vi "Periodic Tasks.vi"(8 "error in":errorcluster) -> ()   [LabVIEW 2023]
doc: "This VI runs in parallel to other robot code. It can contain as many user-defined periodic loops as you need. These can carry out PID or other sorts of timed response."
uses:
  <vilib>/Rock Robotics/WPI/Joystick/XBox Buttons Indexer.ctl
  AimTIFKATS/Implementation/AimTIFKATS Operations.ctl
  Undertake/Implementation/Undertake Operations.ctl
  TIFKATS/Implementation/TIFKATS Operations.ctl
  <vilib>/Rock Robotics/WPI/Utilities/WPI_GetSetVariantRefNum.vi
  <vilib>/Rock Robotics/Network Tables/NT Write Boolean.vi
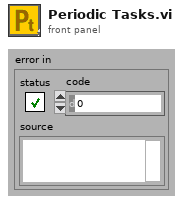
[diagram p1: front panel]
types:
  T1 = typedef "WPI_JoystickDevRef.ctl" = cluster{"Device":T2}
  T2 = typedef "WPI_JoystickDeviceEnum.ctl" = enum16{"USB 0", "USB 1", "USB 2", "USB 3", "USB 4", "USB 5"}
  T3 = typedef "XBox Buttons Indexer.ctl" = enum16{"A", "B", "X", "Y", "Left Bumper", "Right Bumper", "Back", "Start", "Left Joystick", "Right Joystick"}
  T4 = typedef "Undertake Operations.ctl" = enum16{"Reserve", "Read Current", "Immediate", "Onn", "Offf", "Reject"}
  T5 = typedef "AimTIFKATS Operations.ctl" = enum16{"Reserve", "Read Current", "Immediate", "Angle up", "Angle down", "Angle to angle", "Stop rotate"}
  T6 = typedef "TIFKATS Operations.ctl" = enum16{"Reserve", "Read Current", "Immediate", "Load", "Shoot", "Intake", "Spit", "Stop All"}
  T7 = typedef "WPI_DigitalInputDevRef.ctl" = cluster{"DevStatus":errorcluster, "DIO Channel":T8}
  T8 = typedef "FPGA_DIOChannel.ctl" = enum8{"DIO 0", "DIO 1", "DIO 2", "DIO 3", "DIO 4", "DIO 5", "DIO 6", "DIO 7", "DIO 8", "DIO 9", "DIO MXP 0", "DIO MXP 1", "DIO MXP 2", "DIO MXP 3", "DIO MXP 4", "DIO MXP 5", "DIO MXP 6", "DIO MXP 7", "DIO MXP 8", "DIO MXP 9", "DIO MXP 10", "DIO MXP 11", "DIO MXP 12", "DIO MXP 13", "DIO MXP 14", "DIO MXP 15", "SPI Port CS1", "SPI Port CS2", "SPI Port CS3", "SPI Port MISO", "SPI Port MOSI", "Invalid"}
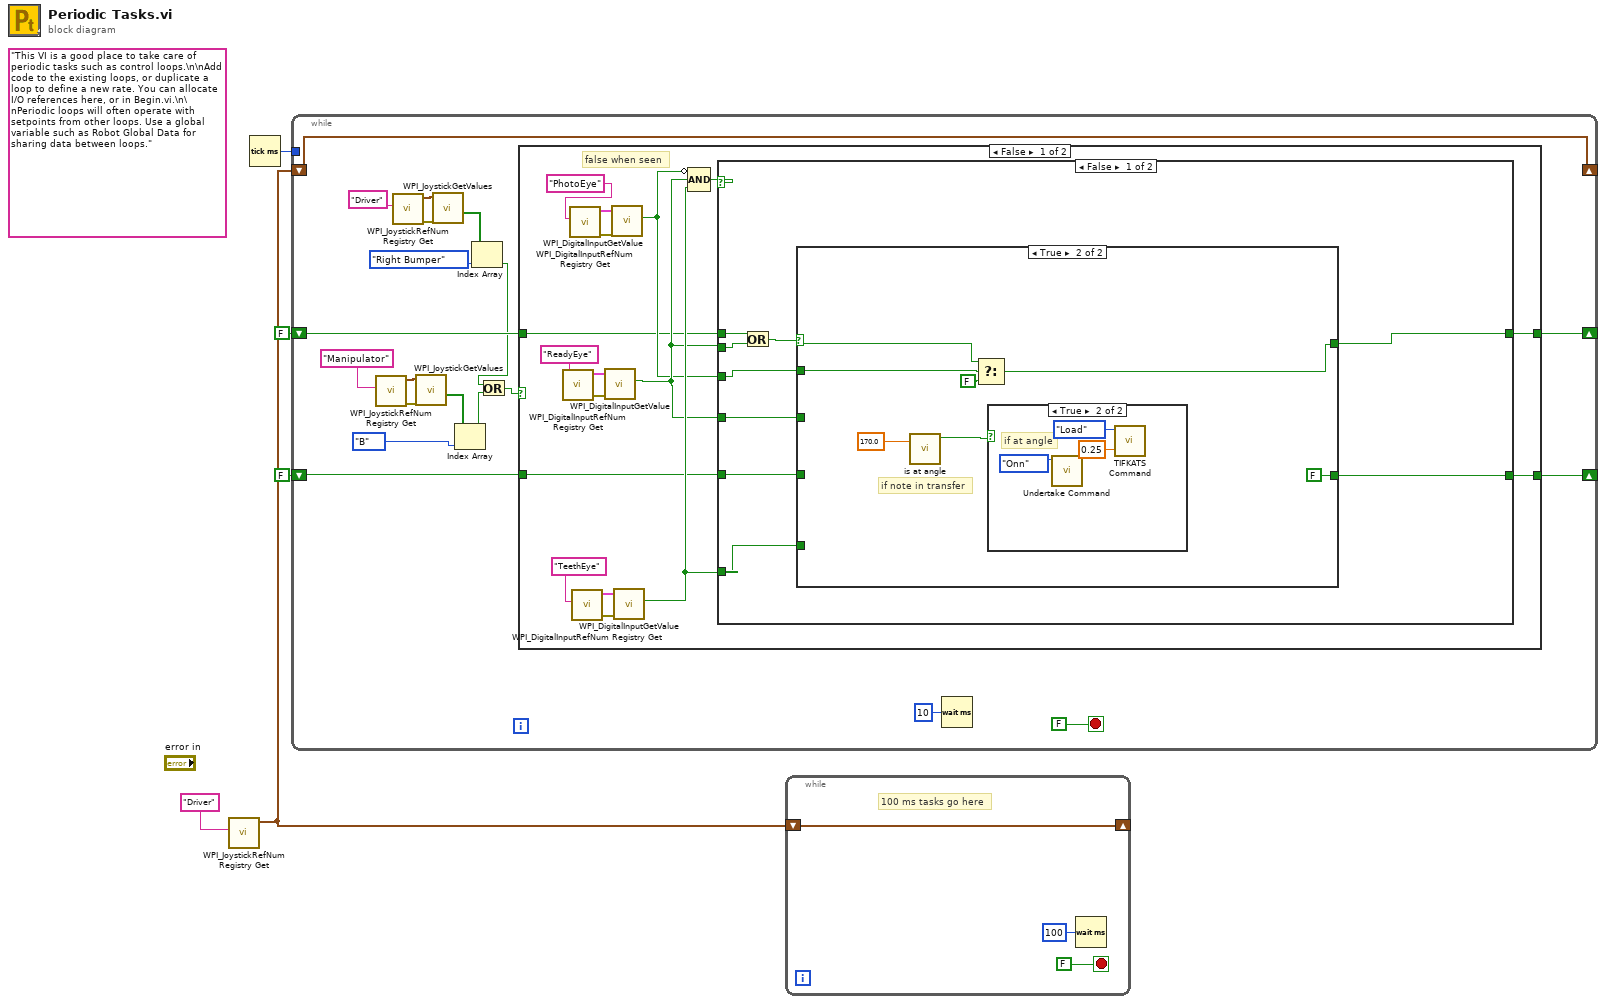
[diagram p0: block diagram]
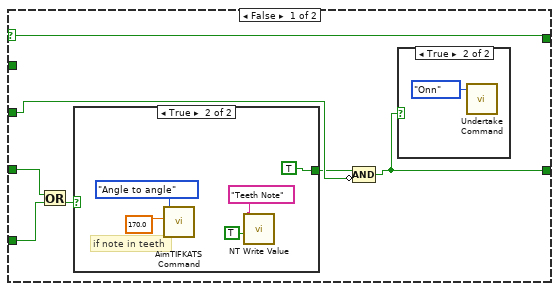
[diagram p2: hidden frame]
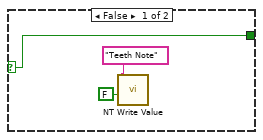
[diagram p4: hidden frame]
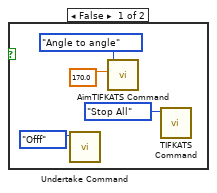
[diagram p5: hidden frame]
diagram:
  (unwired) "This VI is a good place to take care of periodic tasks such as control loops.\n\nAdd code to the existing loops, or duplicate a loop to define a new rate. You can allocate I/O references here, or in Begin.vi.\n\nPeriodic loops will often operate with setpoints from other loops. Use a global variable such as Robot Global Data for sharing data between loops."
  n1 = call <vilib>:"WPI_JoystickRefNum Registry Get.vi"("refnum name"="Driver") -> ("JoystickDevRef"=w4:T1)  [unwired: 1 in, 9 out]
  n2 = Tick Count (ms)() -> (millisecond timer value=w3:u32)
  n3 = while {
    shift-right: [w24] -> _
    shift-left: w4 -> [w24]
    tunnel: w3 -> [_]
    shift-right: [w17] -> _
    shift-left: FALSE -> [w16]
    shift-right: [w14] -> _
    shift-left: FALSE -> [w15]
    stop <- FALSE stop-if-true
    n4 = call <vilib>:"WPI_JoystickRefNum Registry Get.vi"("refnum name"="Manipulator") -> ("error out"=w11:errorcluster, "JoystickDevRef"=w12:T1)  [unwired: 1 in, 8 out]
    n5 = call <vilib>:"WPI_JoystickRefNum Registry Get.vi"("refnum name"="Driver") -> ("error out"=w20:errorcluster, "JoystickDevRef"=w21:T1)  [unwired: 1 in, 8 out]
    n6 = call <vilib>:"WPI_JoystickGetValues.vi"("error in (no error)"=w11, "JoystickDevRef"=w12) -> ("Buttons"=w9:bool[])  [unwired: 5 in, 4 out]
    n7 = call <vilib>:"WPI_JoystickGetValues.vi"("error in (no error)"=w20, "JoystickDevRef"=w21) -> ("Buttons"=w18:bool[])  [unwired: 5 in, 4 out]
    n8 = Index Array(array=w9, index=XBox_Buttons_Indexer."B" ("XBox Buttons")) -> (element=w6:bool)
    n9 = Index Array(array=w18, index=XBox_Buttons_Indexer."Right Bumper" ("XBox Buttons")) -> (element=w7:bool)
    n10 = Or(x=w7, y=w6) -> (x .or. y?=w8:bool)
    n11 = case shown="False" w8 {
      tunnel: [w31 w85] -> w17
      tunnel: w16 -> [w30 w85]
      tunnel: w15 -> [w27 w84]
      tunnel: [w26 w84] -> w14
      frame False {
        # "false when seen"
        n12 = call <vilib>:"WPI_DigitalInputRefNum Registry Get.vi"("refnum name"="ReadyEye") -> ("error out"=w42:errorcluster, "DigitalInputDevRef"=w41:T7)  [unwired: 9 in]
        n13 = call <vilib>:"WPI_DigitalInputRefNum Registry Get.vi"("refnum name"="PhotoEye") -> ("error out"=w37:errorcluster, "DigitalInputDevRef"=w38:T7)  [unwired: 9 in]
        n14 = call <vilib>:"WPI_DigitalInputRefNum Registry Get.vi"("refnum name"="TeethEye") -> ("error out"=w39:errorcluster, "DigitalInputDevRef"=w40:T7)  [unwired: 9 in]
        n15 = call <vilib>:"WPI_DigitalInputGetValue.vi"("error in (no error)"=w42, "DigitalInputDevRef"=w41) -> ("Value"=w29:bool)  [unwired: 7 in, 2 out]
        n16 = call <vilib>:"WPI_DigitalInputGetValue.vi"("error in (no error)"=w37, "DigitalInputDevRef"=w38) -> ("Value"=w28:bool)  [unwired: 7 in, 2 out]
        n17 = call <vilib>:"WPI_DigitalInputGetValue.vi"("error in (no error)"=w39, "DigitalInputDevRef"=w40) -> ("Value"=w32:bool)  [unwired: 7 in, 2 out]
        n18 = Compound Arithmetic op=AND(invert w28, w29, w32) -> (w33:bool)
        n19 = case shown="False" w33 {
          tunnel: w32 -> [w51 _]
          tunnel: w29 -> [w46 _]
          tunnel: w29 -> [w50 _]
          tunnel: [w49 w83] -> w31
          tunnel: w30 -> [w48 w83]
          tunnel: w28 -> [w43 _]
          tunnel: w27 -> [w47 w82]
          tunnel: [w44 w82] -> w26
          frame False {
            n20 = Or(x=w47, y=w46) -> (x .or. y?=w45:bool)
            n21 = case shown="True" w45 {
              selector: w45 -> [w52 w70]
              tunnel: w51 -> [w58 _]
              tunnel: w50 -> [w55 _]
              tunnel: [w53 FALSE] -> w49
              tunnel: w48 -> [w56 _]
              tunnel: [w52 w69] -> w44
              tunnel: w43 -> [_ w71]
              frame False {
                n22 = Or(x=w56, y=w58) -> (x .or. y?=w57:bool)
                n23 = case shown="True" w57 {
                  selector: w57 -> [w60 _]
                  tunnel: [w60 TRUE] -> w54
                  frame False {
                    n24 = call-poly <vilib>:"NT Write Value.vi"("value"=FALSE, "name"="Teeth Note") -> ()  [unwired: 9 in, 1 out]
                  }
                  frame True {
                    # "if note in teeth"
                    n25 = call "AimTIFKATS Command.vi"("Operation"=AimTIFKATS_Operations."Angle to angle", "Setpoint"=170.0) -> ()  [unwired: 8 in, 1 out]
                    n26 = call-poly <vilib>:"NT Write Value.vi"("value"=TRUE, "name"="Teeth Note") -> ()  [unwired: 9 in, 1 out]
                  }
                }
                n27 = Compound Arithmetic op=AND(w54, invert w55) -> (w53:bool)
                n28 = case shown="True" w53 {
                  frame False {
                  }
                  frame True {
                    n29 = call "Undertake Command.vi"("Operation"=Undertake_Operations."Onn") -> ()  [unwired: 9 in, 1 out]
                  }
                }
              }
              frame True {
                # "if note in transfer"
                n30 = call "is at angle.vi"("x"=170.0) -> ("In Range?"=w72:bool)  [unwired: 10 in]
                n31 = Select(t=w70, s=w71, f=FALSE) -> (s? t:f=w69:bool)
                n32 = case shown="True" w72 {
                  frame False {
                    n33 = call "Undertake Command.vi"("Operation"=Undertake_Operations."Offf") -> ()  [unwired: 9 in, 1 out]
                    n34 = call "AimTIFKATS Command.vi"("Operation"=AimTIFKATS_Operations."Angle to angle", "Setpoint"=170.0) -> ()  [unwired: 8 in, 1 out]
                    n35 = call "TIFKATS Command.vi"("Operation"=TIFKATS_Operations."Stop All") -> ()  [unwired: 10 in, 1 out]
                  }
                  frame True {
                    # "if at angle"
                    n36 = call "Undertake Command.vi"("Operation"=Undertake_Operations."Onn") -> ()  [unwired: 9 in, 1 out]
                    n37 = call "TIFKATS Command.vi"("Setpoint"=0.25, "Operation"=TIFKATS_Operations."Load") -> ()  [unwired: 9 in, 1 out]
                  }
                }
              }
            }
          }
          frame True {
            # "if no note in robot"
          }
        }
      }
      frame True {
      }
    }
    n38 = Wait (ms)(milliseconds to wait=u32 10) -> ()  [unwired: 1 out]
  }
  n39 = while {
    shift-right: [w86] -> _
    shift-left: w4 -> [w86]
    stop <- FALSE stop-if-true
    # "100 ms tasks go here"
    n40 = Wait (ms)(milliseconds to wait=u32 100) -> ()  [unwired: 1 out]
  }
